vi "Oscilloscope_Dual_MohammadVersion.vi"() -> ()   [LabVIEW 2024]
uses:
  <vilib>/DAQmx/read.llb/DAQmx Read (Analog 1D Wfm NChan NSamp).vi
  <vilib>/DAQmx/create/channels.llb/DAQmx Create Channel (AI-Voltage-Basic).vi
  <vilib>/DAQmx/configure/timing.llb/DAQmx Timing (Sample Clock).vi
  <vilib>/DAQmx/miscellaneous.llb/DAQmx Fill In Error Info.vi
panel:
  out "right 2":dynamicdata(graph)=[{"t0"=timestamp(3806599236.6321588 s since 1904-01-01), "dt"=4.999999999999579e-07, "Y"=array[202167 elements], "attributes"=variant("NI_ChannelName"=variant(string "cDAQ2Mod1/ai1"), "NI_UnitDescription"=variant(string "Volts"))}]
  out "left 2":dynamicdata(graph)=[{"t0"=timestamp(3806599236.6321588 s since 1904-01-01), "dt"=4.999999999999579e-07, "Y"=array[202167 elements], "attributes"=variant("NI_ChannelName"=variant(string "cDAQ2Mod1/ai0"), "NI_UnitDescription"=variant(string "Volts"))}]
  in  "Stop Visualization":bool
  in  "stop Acquisition":bool
  in  "active edge":i32(ring)=10280 items=["Rising"=10280, "Falling"=10171]
  in  "File (0:open)":T1(ring)
  in  "File Name 2":string
  in  "Folder to save file to 2":path=path "A:/Source Localization/Material Evaluation paper/Dataset/Microphone Characterization/Clean Source"
  in  "physical channels 2":tag="cDAQ2Mod1/ai0, cDAQ2Mod1/ai3"
  in  "Sample Rate 2":dbl=200000.0 format="%0.2f"
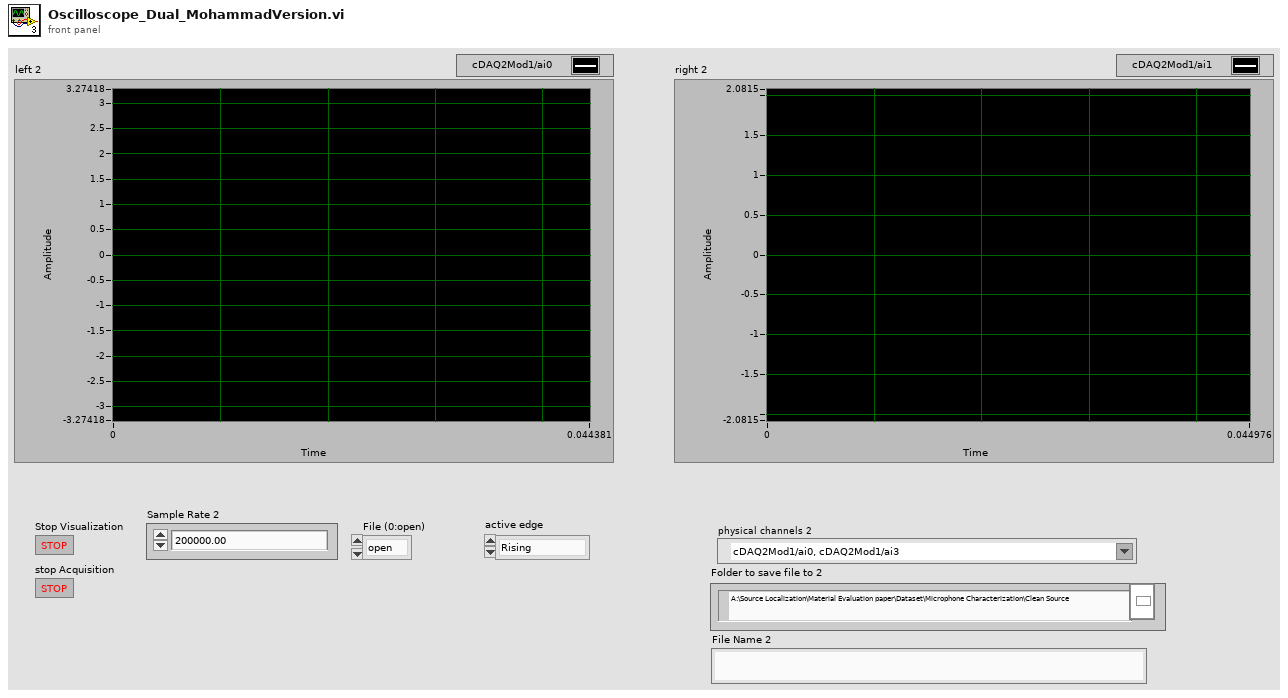
[diagram p1: front panel]
types:
  T1 = enum16{"open", "open or create", "create or replace", "create", "open (read-only)"}
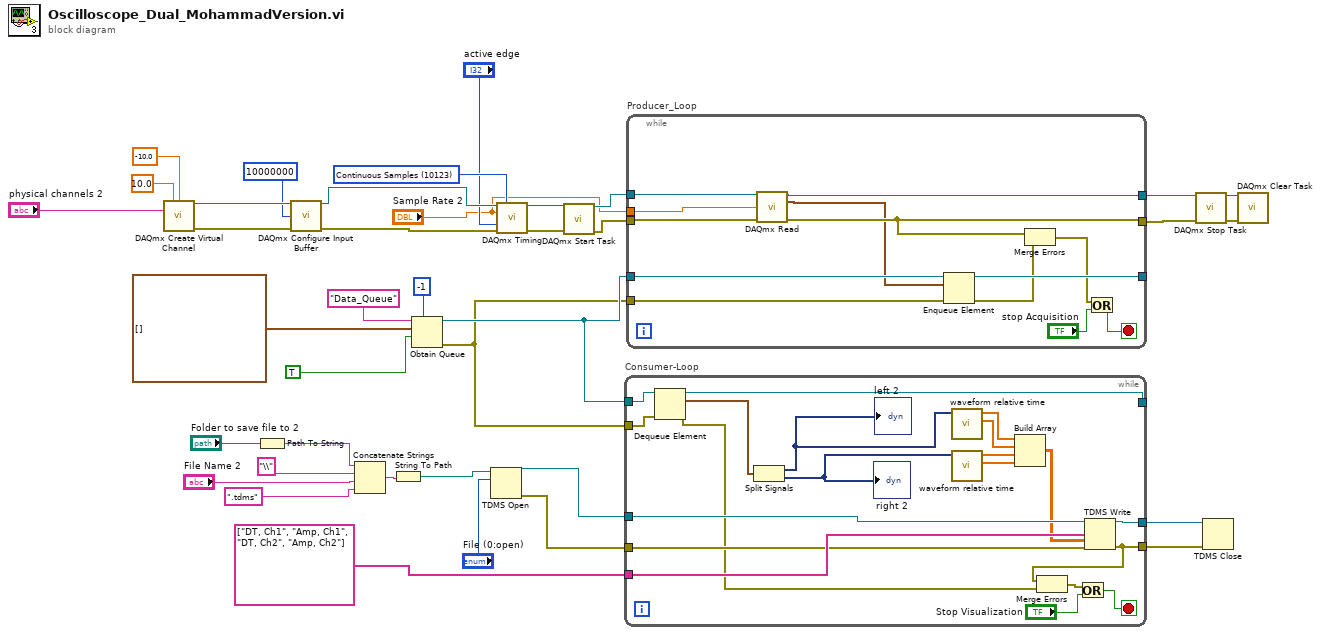
[diagram p0: block diagram]
diagram:
  w33 = 10123 items=["Finite Samples"=10178, "Continuous Samples"=10123, "Hardware Timed Single Point"=12522] ("sample mode")
  n1 = call-poly <vilib>:"DAQmx Create Virtual Channel.vi"("maximum value"=10.0, "minimum value"=-10.0, "physical channels"="physical channels 2") -> ("task out"=w38:refnum<k21>, "error out"=w37:errorcluster)  [unwired: 11 in]
  n2 = Path To String(path="Folder to save file to 2") -> (string=w27:string)
  n3 = call <vilib>:"DAQmx Configure Input Buffer.vi"("task/channels in"=w38, "buffer size (in samples per channel)"=u32 10000000, "error in"=w37) -> ("task out"=w35:refnum<k21>, "error out"=w34:errorcluster)  [unwired: 11 in]
  n4 = Concatenate Strings(w27, "\\" ("string"), "File Name 2", ".tdms" ("string")) -> (w26:string)
  n5 = String To Path(string=w26) -> (path=w23:path)
  n6 = Obtain Queue(max queue size (-1, unlimited)=-1, name (unnamed)="Data_Queue", element data type=waveform(dbl)[] [] ("waveform"), create if not found? (T)=TRUE) -> (queue out=w11:refnum<queue>, error out=w6:errorcluster)  [unwired: 1 in, 1 out]
  n7 = TDMS Open(10:"File (0:open)", 11:w23) -> (0:w9:errorcluster, 3:w10:refnum<k34>)  [unwired: 5 in]
  n8 = call-poly <vilib>:"DAQmx Timing.vi"("task/channels in"=w35, "sample mode"=w33, "rate"="Sample Rate 2", "active edge"="active edge", "error in"=w34) -> ("task out"=w21:refnum<k21>, "error out"=w20:errorcluster)  [unwired: 9 in]
  n9 = call <vilib>:"DAQmx Start Task.vi"("task/channels in"=w21, "error in"=w20) -> ("task out"=w18:refnum<k21>, "error out"=w17:errorcluster)  [unwired: 12 in]
  n10 = while "Consumer-Loop" {
    tunnel: w11 -> [w58]
    tunnel: w10 -> [w55]
    tunnel: w9 -> [w53]
    tunnel: w6 -> [w57]
    tunnel: [w56] -> _
    tunnel: string[] ["DT, Ch1", "Amp, Ch1", "DT, Ch2", "Amp, Ch2"] ("channel name(s) in (Untitled)") -> [w54]
    tunnel: [w40] -> w4
    tunnel: [w39] -> w3
    stop <- w51 stop-if-true
    n11 = Dequeue Element(queue=w58, error in (no error)=w57) -> (queue out=w56:refnum<queue>, element=w49:waveform(dbl)[], error out=w46:errorcluster)  [unwired: 1 in, 1 out]
    n12 = Split Signals(w49) -> (w43:dynamicdata, w42:dynamicdata)  [unwired: 2 in]
    "left 2" <- w43
    "right 2" <- w42
    n13 = call "waveform relative time.vi"("signal in"=w43) -> ("Y"=w44:dbl[], "Relative Time"=w45:dbl[])  [unwired: 7 in, 2 out]
    n14 = call "waveform relative time.vi"("signal in"=w42) -> ("Y"=w48:dbl[], "Relative Time"=w47:dbl[])  [unwired: 7 in, 2 out]
    n15 = Build Array(w45, w44, w47, w48) -> (w41:dbl[][])
    n16 = TDMS Write(0:w55, 7:w54, 9:w41, 11:w53) -> (4:w40:refnum<k34>, 15:w39:errorcluster)  [unwired: 2 in, 2 out]
    n17 = Merge Errors(w39, w46) -> (w52:errorcluster)
    n18 = Or(x=w52, y="Stop Visualization") -> (x .or. y?=w51:bool)
  }
  n19 = while "Producer_Loop" {
    tunnel: w18 -> [w69]
    tunnel: w17 -> [w68]
    tunnel: w11 -> [w71]
    tunnel: w6 -> [w70]
    tunnel: [w67] -> _
    tunnel: [w62] -> w8
    tunnel: [w61] -> w7
    tunnel: "Sample Rate 2" -> [w59]
    stop <- w63 stop-if-true
    n20 = call-poly <vilib>:"DAQmx Read.vi"("task/channels in"=w69, "number of samples per channel"=w59, "error in"=w68) -> ("task out"=w62:refnum<k21>, "data"=w60:waveform(dbl)[], "error out"=w61:errorcluster)  [unwired: 10 in]
    n21 = Enqueue Element(queue=w71, element=w60, error in (no error)=w70) -> (queue out=w67:refnum<queue>, error out=w66:errorcluster)  [unwired: 1 in, 1 out]
    n22 = Merge Errors(w61, w66) -> (w65:errorcluster)
    n23 = Or(x=w65, y="stop Acquisition") -> (x .or. y?=w63:bool)
  }
  n24 = call <vilib>:"DAQmx Stop Task.vi"("task/channels in"=w8, "error in"=w7) -> ("task out"=w16:refnum<k21>, "error out"=w15:errorcluster)  [unwired: 12 in]
  n25 = TDMS Close(8:w3, 11:w4) -> ()  [unwired: 2 out]
  n26 = call <vilib>:"DAQmx Clear Task.vi"("task in"=w16, "error in"=w15) -> ()  [unwired: 13 in, 1 out]
